vi "Generate Map URL (Keith Koch's conflicted copy 2013-05-10).vi"   [LabVIEW 2011]
uses:
  _GlobalVariables&Libraries/ATV Program Global Variables.vi
types:
  T1 = cluster{"X":dbl, "Y":dbl, "Zoom":sgl, "Map Type":string, "Google Maps API Key":string, "Map Refresh Rate (ms)":u32, "Navigation Path Color":u32, "Navigation Path Weight":i32, "URL":string, "Boundary Coordinates":cluster{"Latitude":dbl, "Longitude":dbl}[], "GPS Balloon Character":string, "Boundary Path Color":u32, "Boundary Path Weight":i32, "GPS Balloon Size":string, "GPS Balloon Color":string, "GPS Path Color":u32, "GPS Path Weight":i32, "Disable Google Maps":bool}
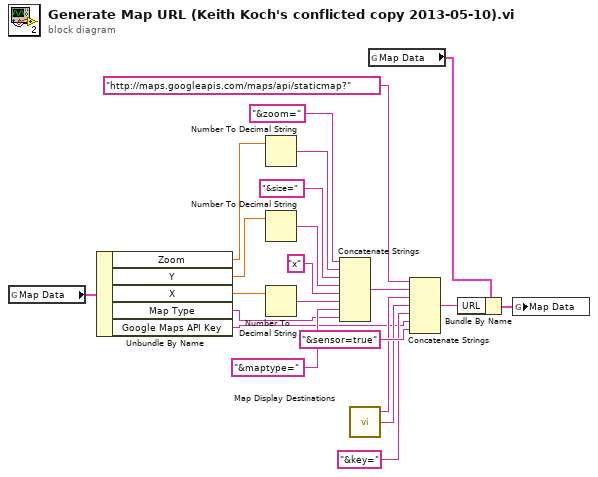
[diagram p0: block diagram]
diagram:
  n1 = global read "ATV Program Global Variables.vi" "Map Data"() -> (w11:T1)
  n2 = Unbundle By Name(w11) -> ("Zoom"=w7:sgl, "Y"=w8:dbl, "X"=w9:dbl, "Map Type"=w10:string, "Google Maps API Key"=w1:string)
  n3 = Number To Decimal String(number=w7) -> (decimal integer string=w21:string)  [unwired: 1 in]
  n4 = Number To Decimal String(number=w8) -> (decimal integer string=w19:string)  [unwired: 1 in]
  n5 = Number To Decimal String(number=w9) -> (decimal integer string=w17:string)  [unwired: 1 in]
  n6 = Concatenate Strings("&zoom=", w21, "&size=", w19, "x", w17, "&maptype=", w10) -> (w15:string)
  n7 = call "Map Display Destinations.vi"() -> ("Navigation Balloon String"=w3:string, "Boundary Path String"=w4:string)  [unwired: 1 out]
  n8 = global read "ATV Program Global Variables.vi" "Map Data"() -> (w14:T1)
  n9 = Concatenate Strings("http://maps.googleapis.com/maps/api/staticmap?" ("string"), w15, w4, w3, "&key=" ("string"), w1, "&sensor=true" ("string")) -> (w13:string)
  n10 = Bundle By Name(cluster=w14, "URL"=w13) -> (w12:T1)
  n11 = global write "ATV Program Global Variables.vi" "Map Data"(w12) -> ()
